vi "Unpack Control Drop.vi"(0 "ControlDropMsg":refnum<class "ControlDropMsg.lvclass">) -> (4 "Ctl Refnum":refnum<vi>, 6 "Control Label":string, 8 "Time":u32, 10 "Coords":T1, 12 "Available Data Names":string[](array[string]), 13 "PlatMods":T2, 14 "Mods":cluster{"Double Click":bool, "Menu Key":bool}, 15 "Button":u16)   [LabVIEW 2017, in "ActorEvents.lvlib" / "ControlDropMsg.lvclass"]
doc: "<License>\nCopyright © 2017 Composed Systems, LLC | All rights reserved\nwww.composed.io\n\nAuthor: Ethan Stern <ethan.stern@composed.io>\n\nThis software is provided \"AS IS\" WITHOUT WARRANTIES, either express or implied, AND IS FOR EDUCATIONAL PURPOSES ONLY.\n</License>"
uses:
  ControlDropMsg.lvclass
  <vilib>/Utility/miscctls.llb/LVPoint32TypeDef.ctl
  ControlDropMsg.lvclass/ControlDropMsg.ctl
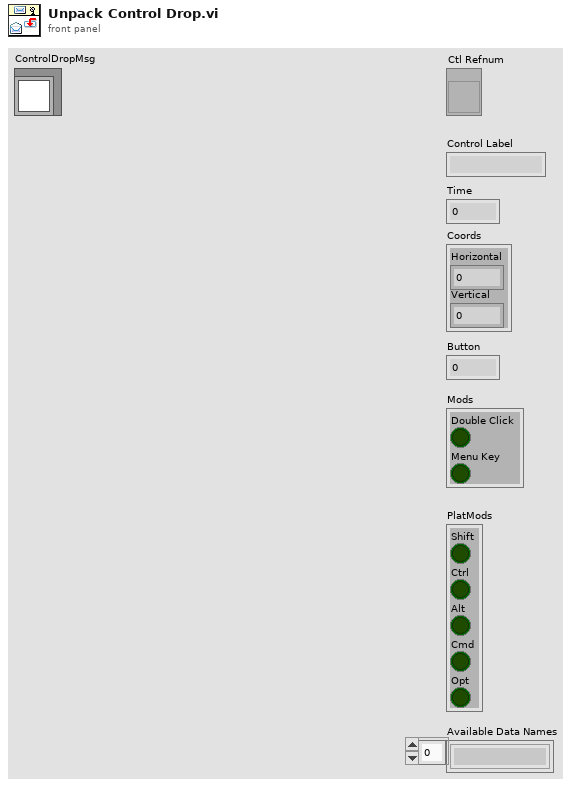
[diagram p1: front panel]
types:
  T1 = typedef "LVPoint32TypeDef.ctl" = cluster{"Horizontal":i32, "Vertical":i32}
  T2 = cluster{"Shift":bool, "Ctrl":bool, "Alt":bool, "Cmd":bool, "Opt":bool}
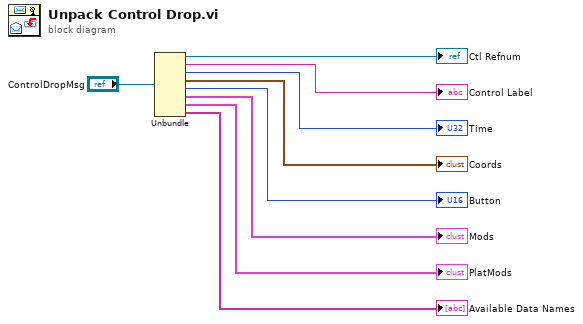
[diagram p0: block diagram]
diagram:
  n1 = Unbundle("ControlDropMsg") -> (→"Ctl Refnum":refnum<vi>, →"Control Label":string, →"Time":u32, →"Coords":T1, →"Button":u16, →"Mods":cluster{"Double Click":bool, "Menu Key":bool}, →"PlatMods":T2, →"Available Data Names":string[])
